vi "Write Text.vi"(5 "Text":refnum<class "Text.lvclass">, 9 "IOName in":refnum<class "IOName.lvclass">) -> (3 "IOName out":refnum<class "IOName.lvclass">)   [LabVIEW 2014, in "IOName.lvclass"]
uses:
  IOName.lvclass
  Text/Text.lvclass
  IOName.lvclass/IOName.ctl
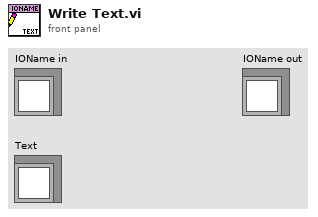
[diagram p1: front panel]
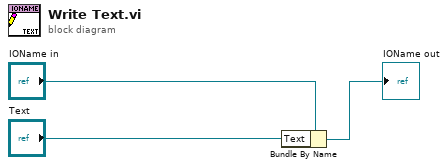
[diagram p0: block diagram]
diagram:
  n1 = Bundle By Name(cluster="IOName in", "Text"="Text") -> (→"IOName out":refnum<class "IOName.lvclass">)
